vi "Send instruction.vi"(8 "error in (no error)":errorcluster, 9 "motor port":u16=5001, 10 "motor ip":string, 11 "instruction":string) -> (0 "error out":errorcluster, 1 "error":bool, 2 "ok":bool, 3 "response":string)   [LabVIEW 2018]
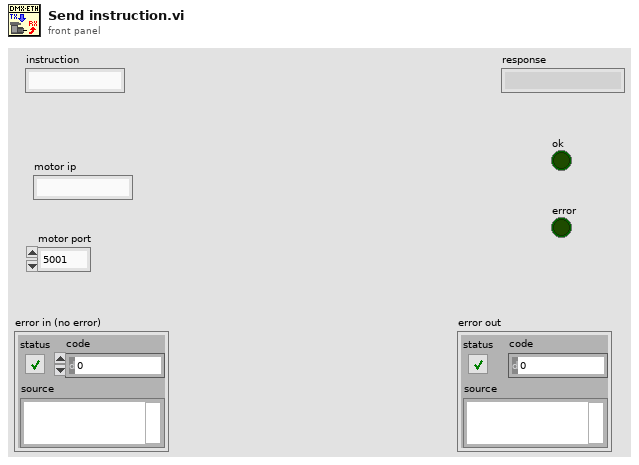
[diagram p1: front panel]
types:
  T1 = enum16{"Standard", "Buffered", "CRLF", "Immediate"}
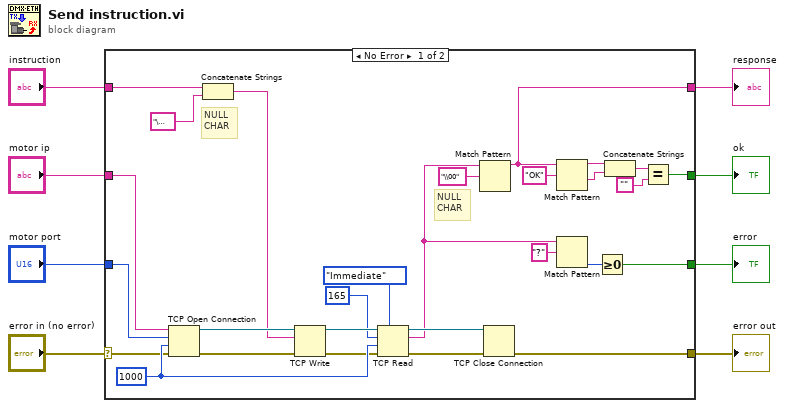
[diagram p0: block diagram]
diagram:
  n1 = case shown="No Error" "error in (no error)" {
    selector: "error in (no error)" -> [w26 w37]
    tunnel: [w18 w37] -> w8
    tunnel: [w23 _] -> w7
    tunnel: "instruction" -> [w17 _]
    tunnel: "motor ip" -> [w29 _]
    tunnel: "motor port" -> [w28 _]
    tunnel: [w19 _] -> w2
    tunnel: [w9 _] -> w1
    frame No Error {
      w30 = 1000 ("timeout ms (60000)")
      # "NULL\nCHAR"
      # "NULL\nCHAR"
      n2 = TCP Open Connection(address=w29, remote port or service name=w28, timeout ms (60000)=w30, error in (no error)=w26) -> (connection ID=w35:refnum<k5>, error out=w36:errorcluster)  [unwired: 1 in]
      n3 = Concatenate Strings(w17, "\u0000" ("search string")) -> (w16:string)
      n4 = TCP Write(connection ID=w35, data in=w16, error in (no error)=w36) -> (connection ID out=w34:refnum<k5>, error out=w14:errorcluster)  [unwired: 1 in, 1 out]
      n5 = TCP Read(connection ID=w34, bytes to read=165, error in (no error)=w14, 7:T1."Immediate" ("mode (standard)"), 9:w30) -> (connection ID out=w32:refnum<k5>, data out=w12:string, error out=w33:errorcluster)
      n6 = Match Pattern(string=w12, regular expression="\\00" ("search string")) -> (before substring=w23:string)  [unwired: 1 in, 3 out]
      n7 = TCP Close Connection(connection ID=w32, error in (no error)=w33) -> (error out=w18:errorcluster)  [unwired: 1 in, 1 out]
      n8 = Match Pattern(string=w23, regular expression="OK" ("y")) -> (before substring=w22:string, after substring=w13:string)  [unwired: 1 in, 2 out]
      n9 = Match Pattern(string=w12, regular expression="?") -> (offset past match=w10:i32)  [unwired: 1 in, 3 out]
      n10 = Greater Or Equal To 0?(x=w10) -> (x >= 0?=w9:bool)
      n11 = Concatenate Strings(w22, w13) -> (w21:string)
      n12 = Equal?(x=w21, y="") -> (x = y?=w19:bool)
    }
    frame Error {
    }
  }
  "error out" <- w8
  "response" <- w7
  "ok" <- w2
  "error" <- w1
